vi "image_to_openai_img_format.vi"(8 "error in (no error)":errorcluster, 11 "imagepaths":path[](array[path])) -> (0 "error out":errorcluster, 3 "image_data":string[](array[string]))   [LabVIEW 2020, in "llm_openai_chatmodels.lvclass"]
uses:
  llm_openai_chatmodels.lvclass
  <vilib>/httpClient/LabVIEWHTTPClient.lvlib
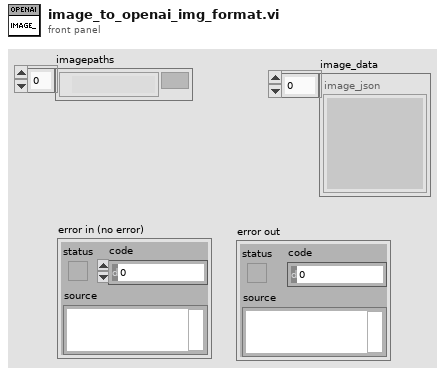
[diagram p1: front panel]
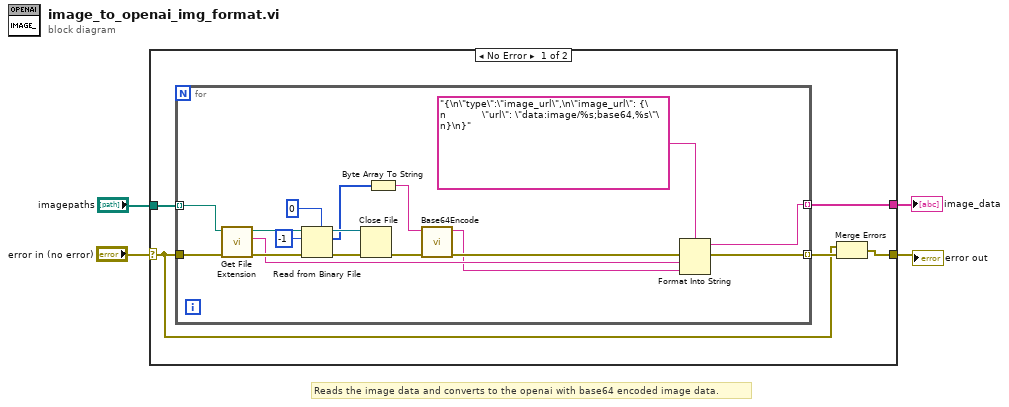
[diagram p0: block diagram]
diagram:
  # "Reads the image data and converts to the openai with base64 encoded image data."
  n1 = case shown="No Error" "error in (no error)" {
    selector: "error in (no error)" -> [w5 w27]
    tunnel: [w9 _] -> w4
    tunnel: "imagepaths" -> [w8 _]
    tunnel: [w6 w27] -> w2
    frame No Error {
      n2 = for {
        tunnel: [w13] -> w9 mode=indexing
        tunnel: w8 -> [w20] mode=indexing
        tunnel: [w15] -> w7 mode=indexing
        tunnel: w5 -> [w19]
        n3 = call <vilib>:"Get File Extension.vi"("error in (no error)"=w19, "file"=w20) -> ("error out"=w26:errorcluster, "lowercase file extension"=w11:string, "dup file"=w25:path)  [unwired: 5 in, 2 out]
        n4 = Read from Binary File(5:u8 0 ("unsigned 8bit integer"), 8:w26, 10:-1 ("count (1)"), 11:w25) -> (0:w23:errorcluster, 2:w17:u8[], 3:w24:refnum<file>)  [unwired: 2 in, 1 out]
        n5 = Close File(refnum=w24, error in=w23) -> (error out=w16:errorcluster)  [unwired: 1 out]
        n6 = Byte Array To String(unsigned byte array=w17) -> (string=w18:string)
        n7 = call <vilib>:"Base64Encode.vi"("error in (no error)"=w16, "buffer in"=w18) -> ("error out"=w12:errorcluster, "encoded string"=w10:string)  [unwired: 8 in]
        n8 = Format Into String(format string="{\n\"type\":\"image_url\",\n\"image_url\": {\n            \"url\": \"data:image/%s;base64,%s\"\n}\n}", error in=w12, w11, w10) -> (resulting string=w13:string, error out=w15:errorcluster)  [unwired: 1 in]
      }
      n9 = Merge Errors(w5, w7) -> (w6:errorcluster)
    }
    frame Error {
    }
  }
  "image_data" <- w4
  "error out" <- w2
